vi "SubPanel_PowerConfiguration_Rev11.vi"(8 "error in":errorcluster, 10 "VISAPowerInfoInputArray":T1(array[cluster]), 11 "DCPowerInformationClusterArray_Input":T3(array[cluster])) -> (0 "error out":errorcluster, 2 "VISAPowerInfoOutputArray":T1(array[cluster]), 3 "DCPowerInformationClusterArray_Output":T3(array[cluster]))   [LabVIEW 2019]
panel:
  out "VISAPowerInformationClusterArray":T1(array[cluster])
  out "DCPowerInformationClusterArray":T2(array[cluster])
  out "VISAPowerInformationClusterOutput":T4(array[cluster])
  in  "VISAPowerInformationClusterInput":T4(array[cluster])
  in  "Exit SubVI":bool
  in  "Instrument Cards (Must Reconfigure if you add new cards or change the names in NI Max)":T5(tab)=enum."PXIe-4139"
  in  "VISA resource name":refnum<visa-resource-name>
  in  "Apply Power Settings":bool
  out "POWER STATUS":bool
  in  "POWER ON":bool
  in  "Voltage Channel 1":dbl
  in  "Voltage Channel 2":dbl
  in  "Voltage Channel 3":dbl
  in  "Current Limit Channel 1":dbl
  in  "Current Limit Channel 2":dbl
  in  "Current Limit Channel 3":dbl
  out "Parameter Configuration Echo":string[][](array[string])
  out "Configuration Echo":string
  in  "Which Channels to Parallelize":u16(ring) items=["I1+I2", "ALL", "I2+I3"]
  in  "Combination Scheme":u16(ring) items=["OFF", "SERIES", "PARALLEL"]
  in  "voltage level channel 0":dbl format="%.6p"
  in  "voltage level channel 1":dbl format="%.6p"
  in  "voltage level channel 2":dbl format="%.6p"
  in  "voltage level channel 3":dbl format="%.6p"
  in  "voltage level channel 4":dbl format="%.6p"
  in  "voltage level channel 5":dbl format="%.6p"
  in  "voltage level channel 6":dbl format="%.6p"
  in  "voltage level channel 7":dbl format="%.6p"
  in  "voltage level channel 8":dbl format="%.6p"
  in  "voltage level channel 9":dbl format="%.6p"
  in  "voltage level channel 10":dbl format="%.6p"
  in  "voltage level channel 11":dbl format="%.6p"
  in  "voltage level channel 12":dbl format="%.6p"
  in  "voltage level channel 13":dbl format="%.6p"
  in  "voltage level channel 14":dbl format="%.6p"
  in  "voltage level channel 15":dbl format="%.6p"
  in  "voltage level channel 16":dbl format="%.6p"
  in  "voltage level channel 17":dbl format="%.6p"
  in  "voltage level channel 18":dbl format="%.6p"
  in  "voltage level channel 19":dbl format="%.6p"
  in  "voltage level channel 20":dbl format="%.6p"
  in  "voltage level channel 21":dbl format="%.6p"
  in  "voltage level channel 22":dbl format="%.6p"
  in  "voltage level channel 23":dbl format="%.6p"
  in  "Active Channel 0":bool
  in  "Active Channel 1":bool
  in  "Active Channel 2":bool
  in  "Active Channel 3":bool
  in  "Active Channel 4":bool
  in  "Active Channel 5":bool
  in  "Active Channel 6":bool
  in  "Active Channel 7":bool
  in  "Active Channel 8":bool
  in  "Active Channel 9":bool
  in  "Active Channel 10":bool
  in  "Active Channel 11":bool
  in  "Active Channel 12":bool
  in  "Active Channel 13":bool
  in  "Active Channel 14":bool
  in  "Active Channel 15":bool
  in  "Active Channel 16":bool
  in  "Active Channel 17":bool
  in  "Active Channel 18":bool
  in  "Active Channel 19":bool
  in  "Active Channel 20":bool
  in  "Active Channel 21":bool
  in  "Active Channel 22":bool
  in  "Active Channel 23":bool
  in  "Channel Name 0":string="NULL0"
  in  "Channel Name 1":string="1p8V_supply"
  in  "Channel Name 2":string="NULL2"
  in  "Channel Name 3":string="NULL3"
  in  "Channel Name 4":string="NULL4"
  in  "Channel Name 5":string="NULL5"
  in  "Channel Name 6":string="NULL6"
  in  "Channel Name 7":string="NULL7"
  in  "Channel Name 8":string="NULL8"
  in  "Channel Name 9":string="NULL9"
  in  "Channel Name 10":string="NULL10"
  in  "Channel Name 11":string="NULL11"
  in  "Channel Name 12":string="NULL12"
  in  "Channel Name 13":string="NULL13"
  in  "Channel Name 14":string="NULL14"
  in  "Channel Name 15":string="NULL15"
  in  "Channel Name 16":string="NULL16"
  in  "Channel Name 17":string="NULL17"
  in  "Channel Name 18":string="NULL18"
  in  "Channel Name 19":string="NULL19"
  in  "Channel Name 20":string="NULL20"
  in  "Channel Name 21":string="NULL21"
  in  "Channel Name 22":string="NULL22"
  in  "Channel Name 23":string="NULL23"
  in  "Apply Power Settings":bool
  in  "Aperture Time (s)":dbl=0.0001
  in  "Measure Record Length":i32=1000000
  in  "current limit (A)":dbl=0.05
  out "All Channel Numbers Array":string[](array[string])=["0", "1", "2", "3", "4", "5", "6", "7", "8", "9", "10", "11", "12", "13", "14", "15", "16", "17", "18", "19", "20", "21", "22", "23"]
  out "Active Channels Indicator":bool[](array[boolean])
  out "Voltage Array":dbl[](array[numeric])=[1.0, 1.8, 1.2, 1.3, 1.4, 1.5, 1.6, 1.7, 1.8, 1.9, 2.0, 2.1, 2.2, 2.3, 2.4, 2.5, 2.6, 2.7, 2.8, 2.9, 3.0, 3.1, 3.2, 3.3]
  out "Active Channel Numbers Array":string[](array[string])=["1"]
  out "Active Channel Voltage Array":dbl[](array[numeric])=[1.8]
  out "Active Channel Names Array":string[](array[string])=["1p8V_supply"]
  in  "voltage level channel 0":dbl format="%.6p"
  in  "Active Channel 0":bool
  in  "Apply Power Settings":bool
  in  "Channel Name 0":string="1p6_supply"
  out "Active Channel Voltage Array":dbl[](array[numeric])=[1.68]
  out "Active Channels Indicator":bool[](array[boolean])
  out "Voltage Array":dbl[](array[numeric])=[1.68]
  out "Active Channel Names Array":string[](array[string])=["1p6_supply"]
  out "Active Channel Numbers Array":string[](array[string])=["0"]
  out "All Channel Numbers Array":string[](array[string])=["0"]
  in  "current limit (A)":dbl=0.05
  in  "Measure Record Length":i32=1000000
  in  "Aperture Time (s)":dbl=0.001
  out "DCPowerInformationClusterOutput":T6(array[cluster])
  in  "DCPowerInformationClusterInput":T6(array[cluster])
  # "Background Information (Important)\nThis subvi has tabs that allow you to configure different power instruments. There are two options: VISA instruments or DC Power instruments. DC Power instruments are inside of the tester, visa instruments are external. If DCPower instruments are switched out, they will need to be reconfigured within the backend of this code (instructions pending). You are able to identify which channels you want to active, their individual voltage levels and the desired \"name\" of the channel (i.e. if you want channel 0 to be known at the \"ADMV1013_3p3V\" or \"GoodEnough\", you write it here). For the entire instrument, you can determine its capture rate (aperture time) or the current limit. I advise you do NOT alter the \"Measure Record Length\" as this is only if there are issues with the program. Shouldn't ever exceed this value. You apply the settings and they will be echoed back in each tab along with the array above. Multiple instruments can be configured and will show up as separate array elements\n\n\nInstructions (More Important):\n\nSelect instrument of interest (VISA KEITHLEY 2230G-30-6, PXIe-4163, and PXIe-4139 are the ones currently available). \n\n\nFOR DCPOWER INSTRUMENTS (PXI or PXIe)\n\nPress \"Active Channel #\" to select which channels you want to have power applied \n\nType in voltage level in \"Voltage level channel #\"\n\nType in desired channel name in \"Channel Name #\"\n\nType the measurement speed (suggest .0001) in aperture time\n\nType the current limit in \"current limit\"\n\nPress \"Apply Power Settings\" and review the echoed outputs within the tab and in the instrument array above the tabs.\n\nRepeat this process for other instruments\n\n\n\nFOR VISA INSTRUMENTS (NOT PXI or PXIe), note that it is case by case for instruments\n\nSelect resource name (you must know which one it is)\n\nPower on device if using it\n\nApply voltage settings \n\nApply current limits for each channel\n\nSelect which channels you will parallelize if at all\n\nSelect which combination scheme you will apply: OFF (individual channels), SERIES (Channel 1 and 2 in series), PARALLEL (I1 + I2, ALL, I2 + I3)\n\nFOR COMBINATIONS: for a combination scheme you choose, you only apply changes to the first channel of each. example: if you make the system series configuration, you only type you voltage information (i.e. 60V) into channel 1 and the current limit information into channel 1 but channel 3 is still independent of these\n\n\nPress \"Apply Powe Settings\" when complete\n\nReview the echoed values along with the instrument array above"
  # "All Voltage Level Channels are in Volts"
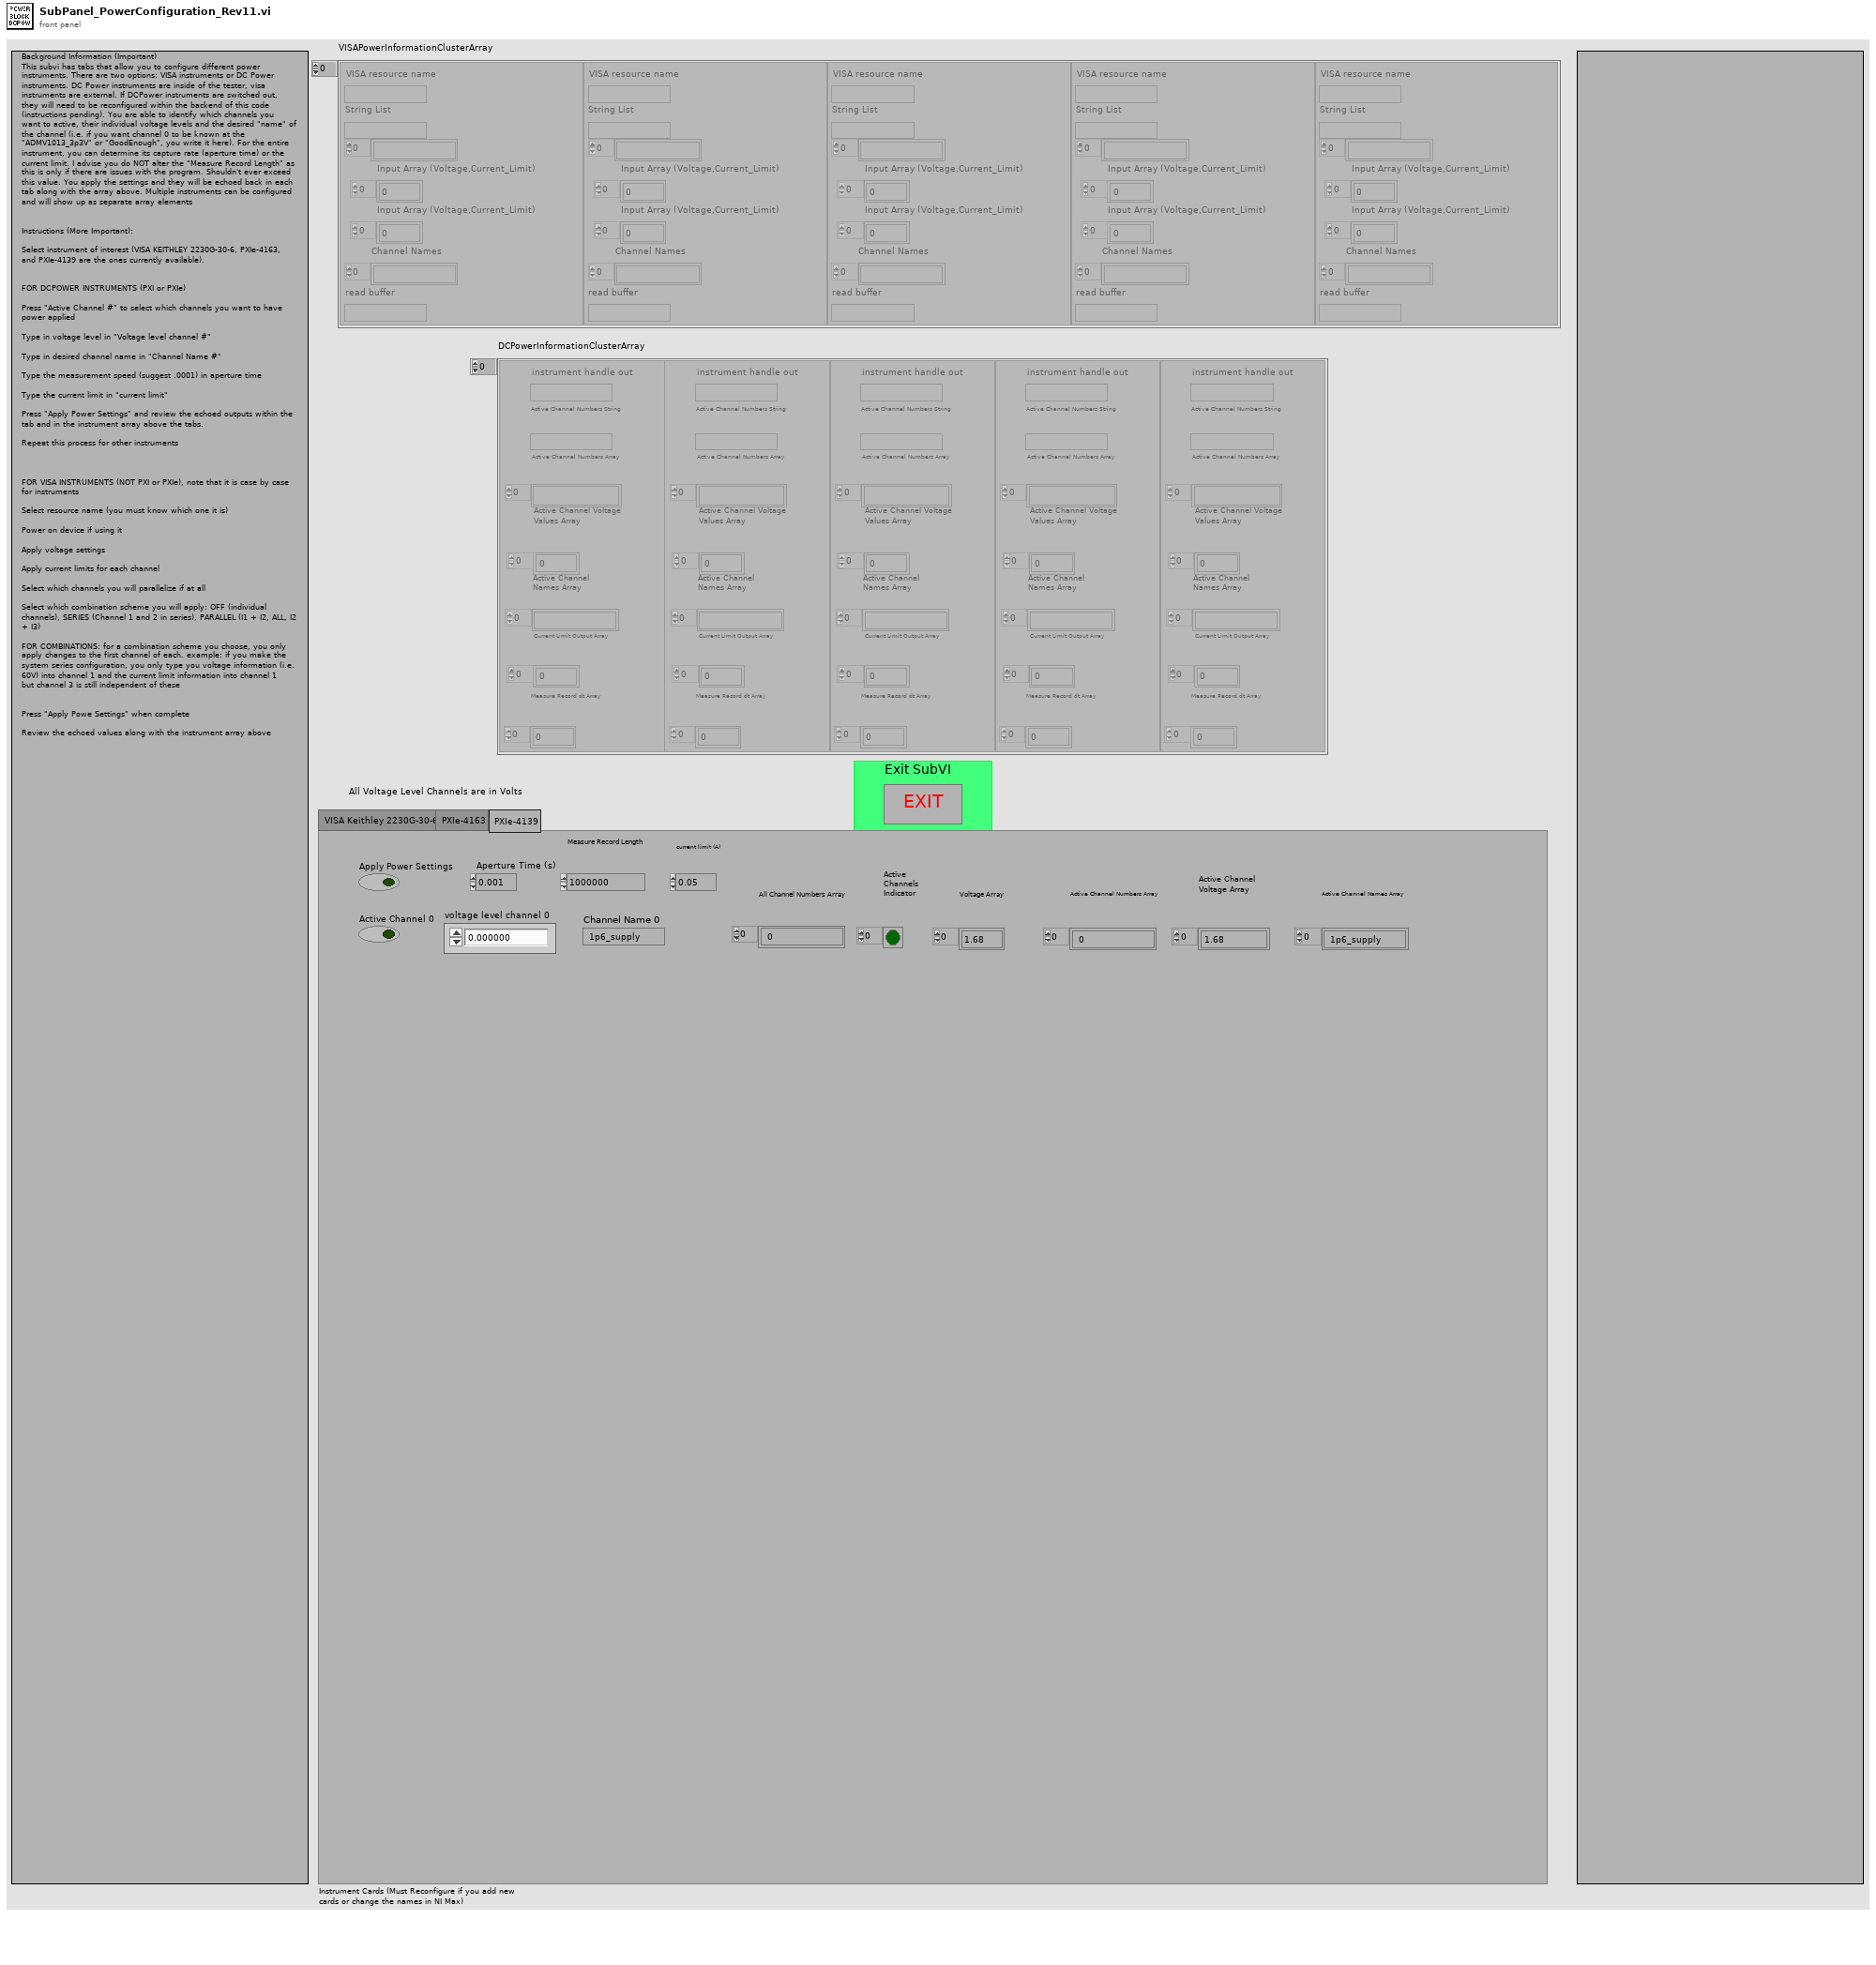
[diagram p1: front panel]
types:
  T1 = cluster{"VISA resource name":refnum<visa-resource-name>, "String List":string, string[], "Input Array (Voltage,Current_Limit)":dbl[], "Input Array (Voltage,Current_Limit)":dbl[], "Channel Names":string[], "read buffer":string}[]
  T2 = cluster{"instrument handle out":refnum<k15>, "Active Channel Numbers String":string, "Active Channel Numbers Array":string[], "Active Channel Voltage Values Array":dbl[], "Active Channel Names Array":string[], "Current Limit Output Array":dbl[], "Measure Record dt Array":dbl[]}[]
  T3 = cluster{"instrument handle out":refnum<k15>, string, string[], dbl[], string[], "Current Limit Output Array":dbl[], dbl[]}[]
  T4 = cluster{"VISA resource name":refnum<visa-resource-name>, "String List":string, string[], "Input Array (Voltage,Current_Limit)":dbl[], "Input Array (Voltage,Current_Limit)":dbl[], "Channel Names":string[]}[]
  T5 = enum32{"VISA Keithley 2230G-30-6", "PXIe-4163", "PXIe-4139"}
  T6 = cluster{"instrument handle out":refnum<k15>, string, string[], dbl[], string[]}[]
  T7 = cluster{"IVI Refnum out":refnum<k15>, "Active Channel Numbers String List":string, "Active Channel Numbers Array":string[], "Active Channel Voltage Array":dbl[], "Active Channel Names Array":string[], "Active Channel Current Limit Array":dbl[], "Active Channel Measure Record Delta Time Array":dbl[]}
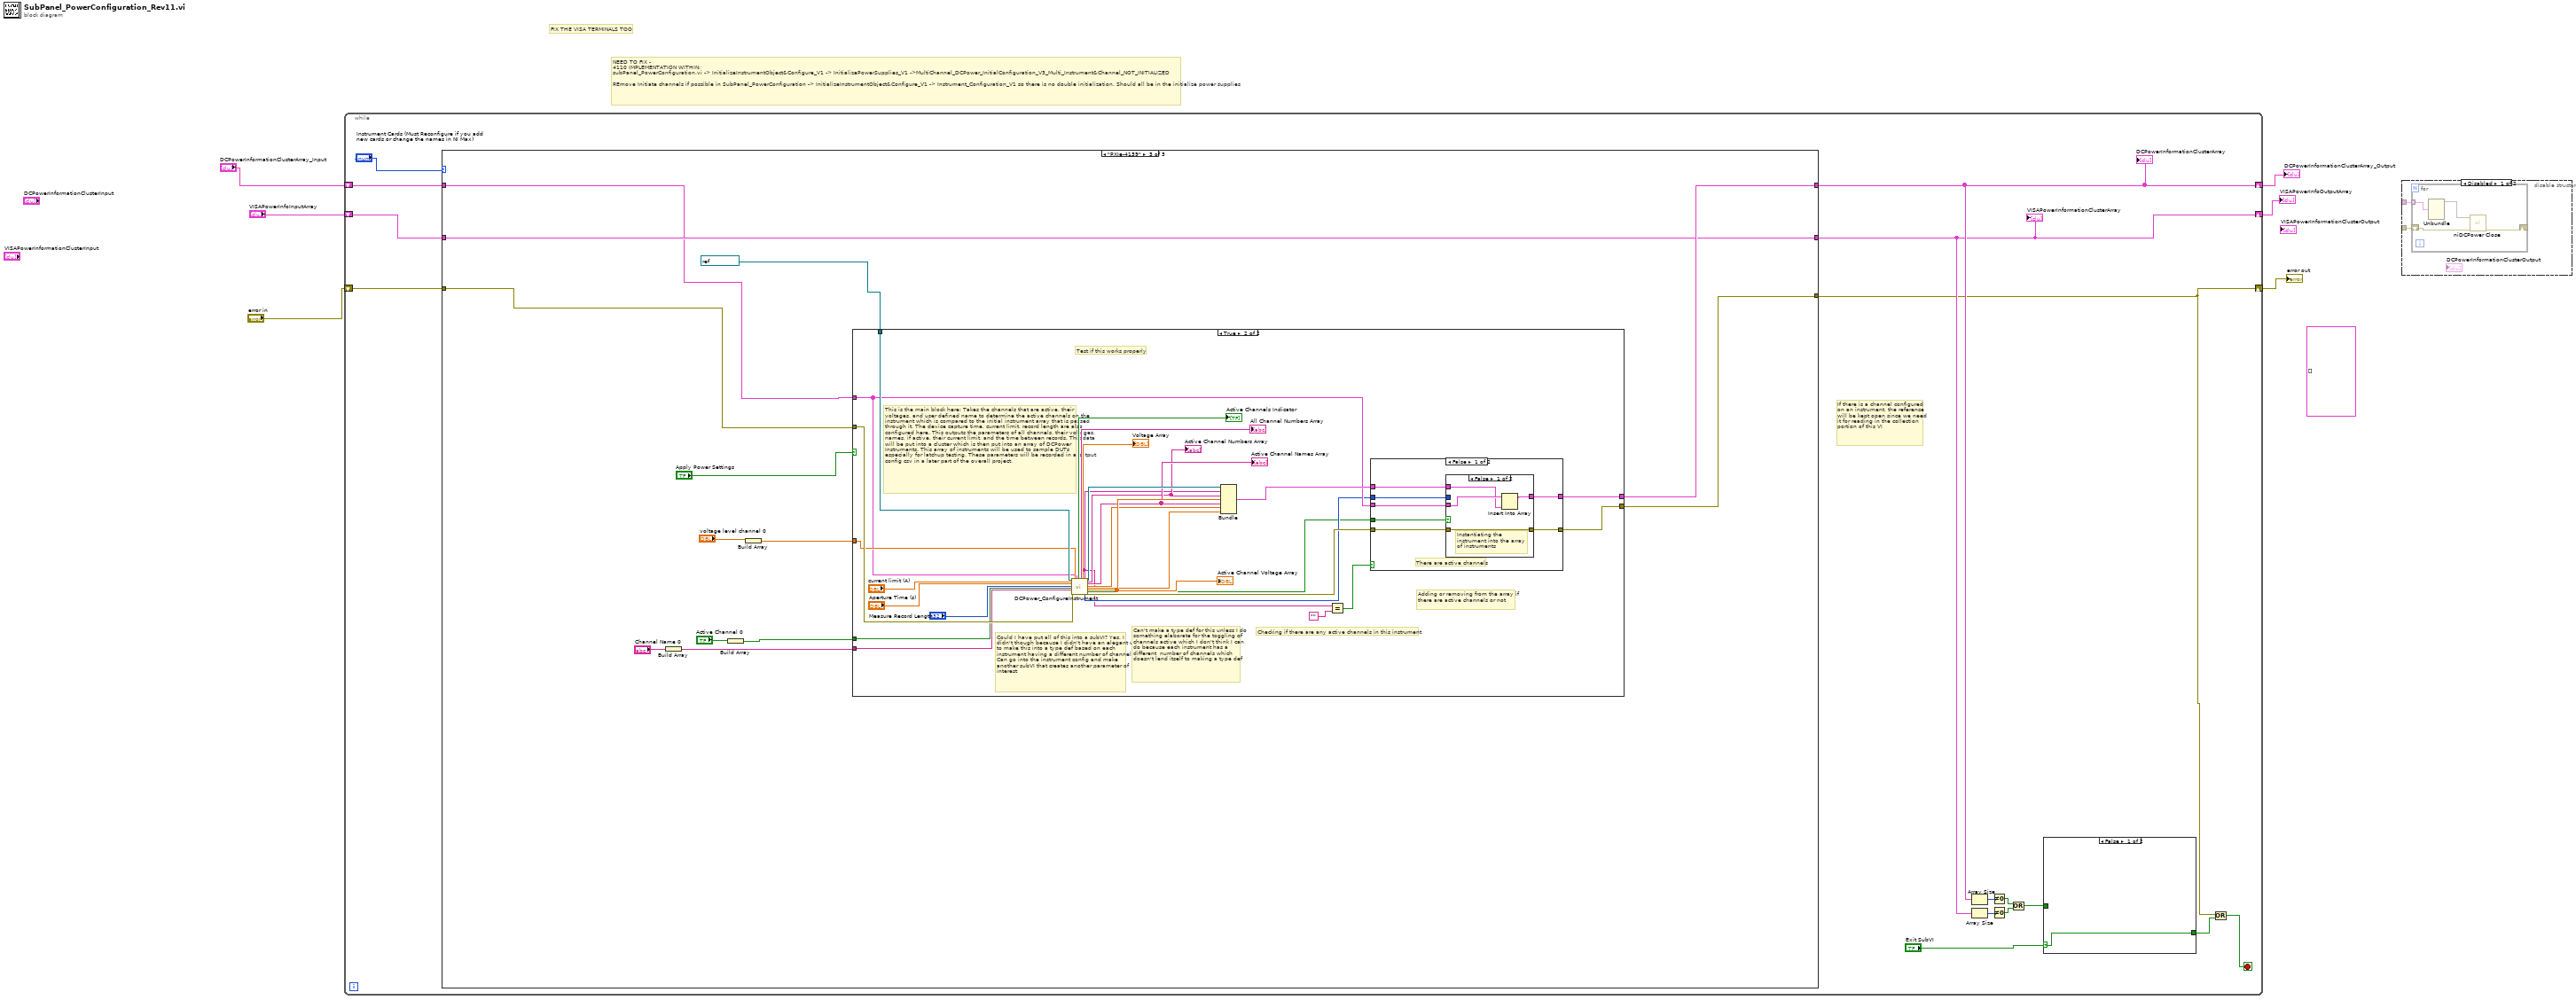
[diagram p0: block diagram]
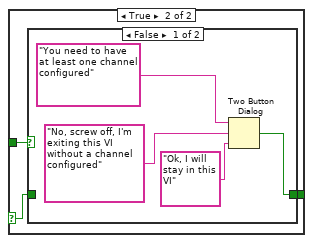
[diagram p3: hidden frame]
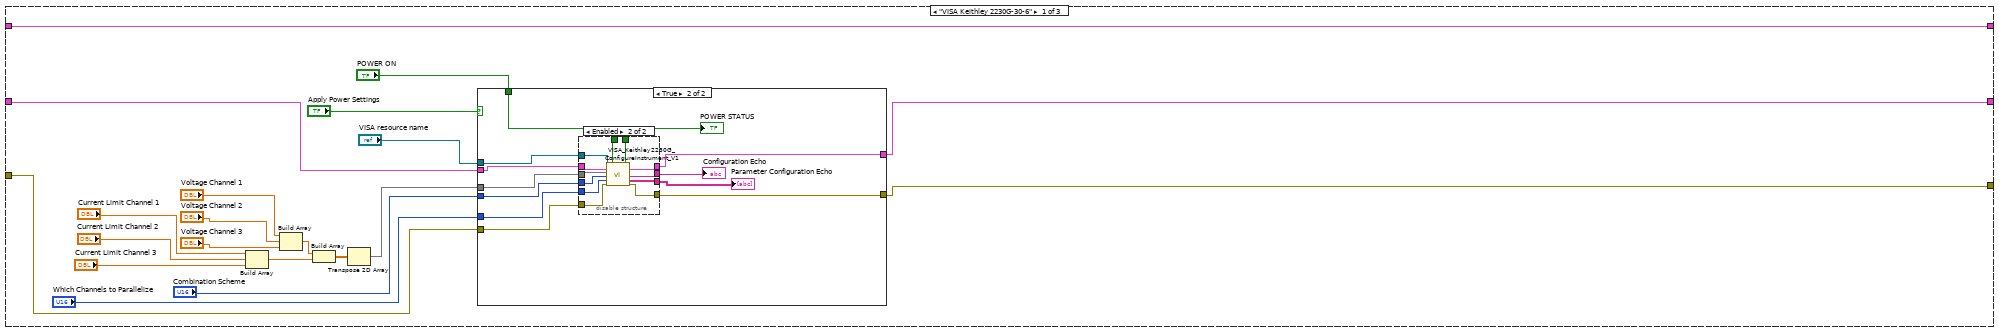
[diagram p5: hidden frame]
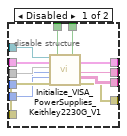
[diagram p7: hidden frame]
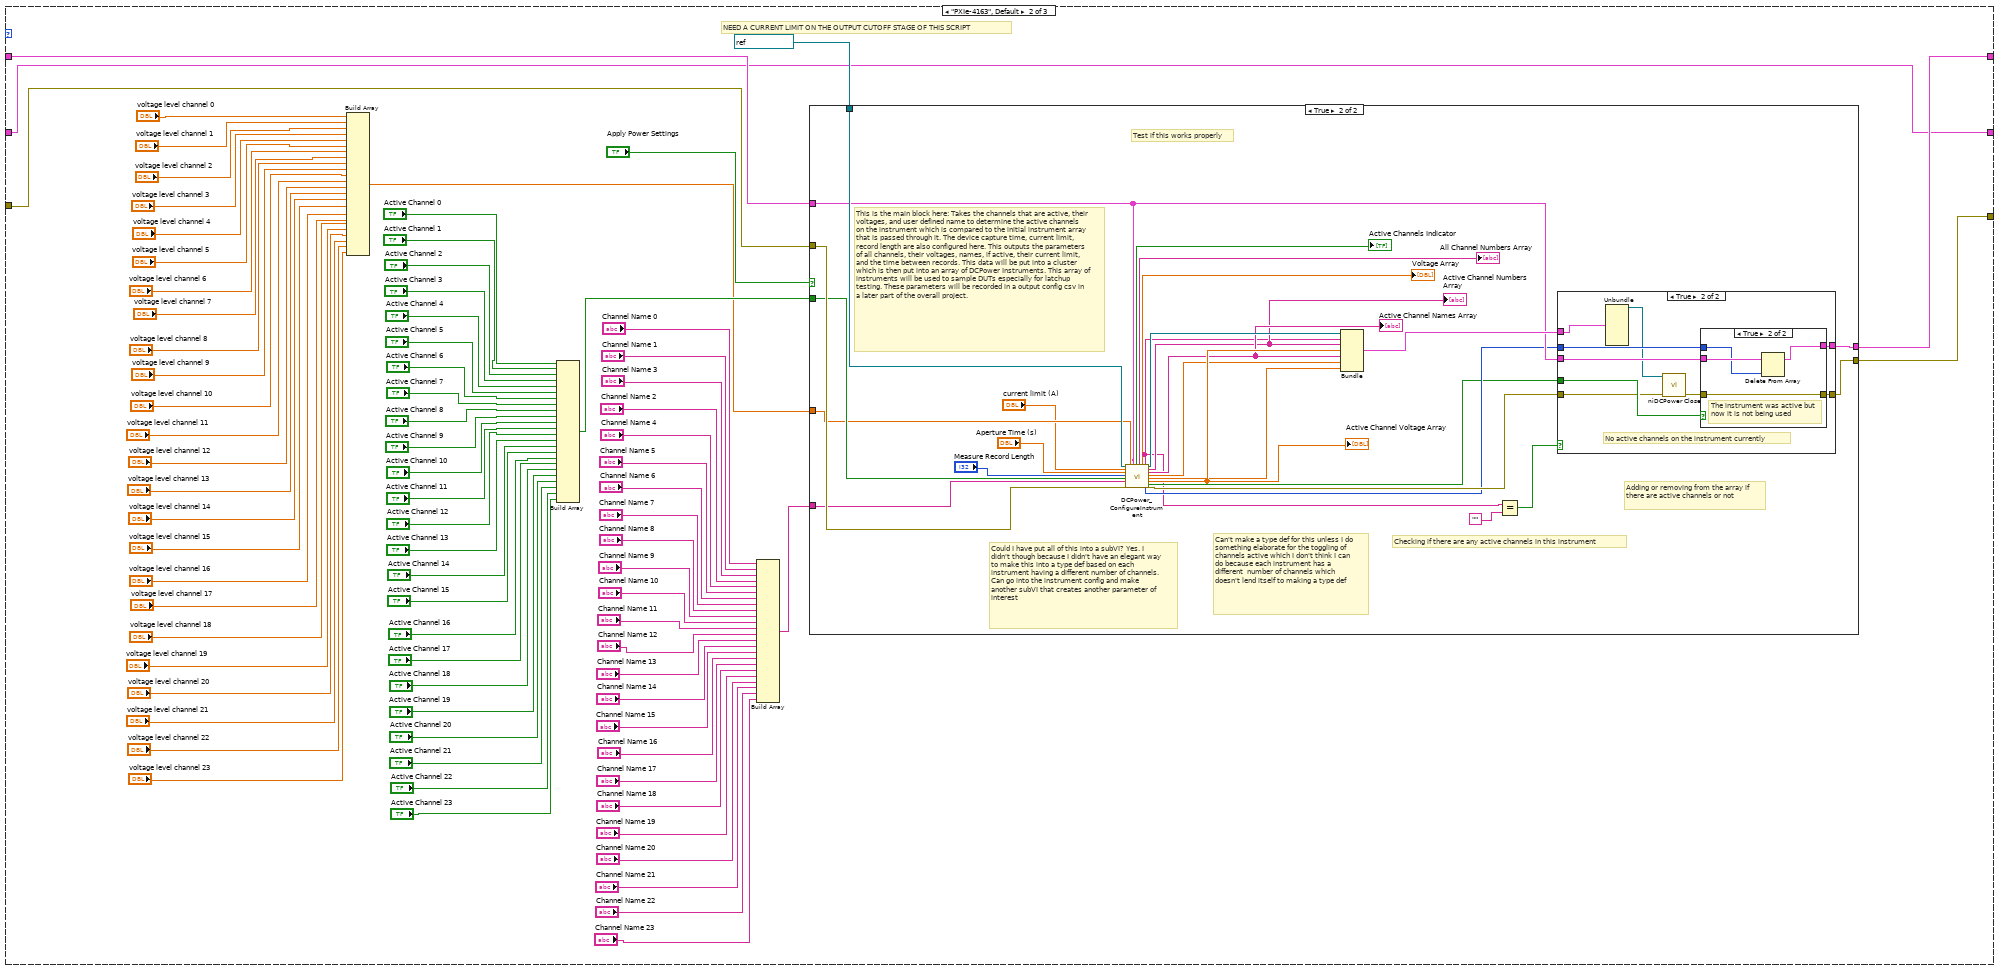
[diagram p8: hidden frame]
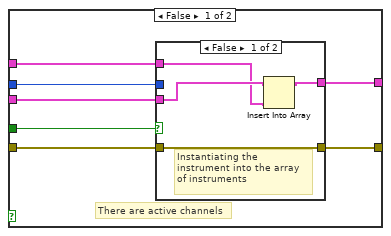
[diagram p10: hidden frame]
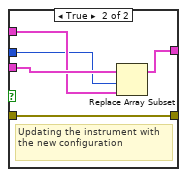
[diagram p11: hidden frame]
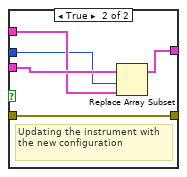
[diagram p14: hidden frame]
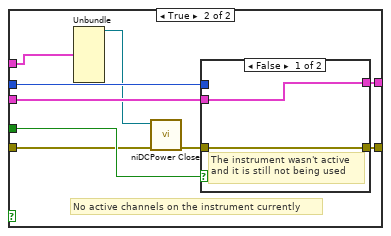
[diagram p15: hidden frame]
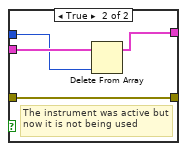
[diagram p16: hidden frame]
diagram:
  (unwired) T3 [] ("DCPowerInformationClusterArray_Input")
  # "FIX THE VISA TERMINALS TOO"
  # "NEED TO FIX - \n4110 IMPLEMENTATION WITHIN:\nsubPanel_PowerConfiguration.vi -> InitializeInstrumentObject&Configure_V1 -> InitializePowerSupplies_V1 ->MultiChannel_DCPower_InitialConfiguration_V3_Multi_Instrument&Channel_NOT_INITIALIZED\n\nREmove Initiate channels if possible in SubPanel_PowerConfiguration -> InitializeInstrumentObject&Configure_V1 -> Instrument_Configuration_V1 so there is no double initialization. Should all be in the initialize power supplies"
  n1 = while {
    shift-right: [w17] -> w1
    shift-left: "DCPowerInformationClusterArray_Input" -> [w21]
    shift-right: [w9] -> w5
    shift-left: "error in" -> [w20]
    shift-right: [w16] -> w3
    shift-left: "VISAPowerInfoInputArray" -> [w18]
    stop <- w7 stop-if-true
    # "If there is a channel configured on an instrument, the reference will be kept open since we need it for reading in the collection portion of this VI"
    n2 = case shown="\"PXIe-4139\"" "Instrument Cards (Must Reconfigure if you add new cards or change the names in NI Max)" {
      tunnel: w21 -> [w47 w97 w231]
      tunnel: w20 -> [w35 w93 w239]
      tunnel: [w32 w92 w233] -> w9
      tunnel: [w47 w91 w234] -> w17
      tunnel: w18 -> [w48 w90 w232]
      tunnel: [w31 w90 w232] -> w16
      frame "VISA Keithley 2230G-30-6" {
        n3 = Build Array("Current Limit Channel 1", "Current Limit Channel 2", "Current Limit Channel 3") -> (w45:dbl[])
        n4 = Build Array("Voltage Channel 1", "Voltage Channel 2", "Voltage Channel 3") -> (w44:dbl[])
        n5 = Build Array(w44, w45) -> (w46:dbl[][])
        n6 = Transpose 2D Array(2D array=w46) -> (transposed array=w36:dbl[][])
        n7 = case shown="True" "Apply Power Settings" {
          tunnel: "VISA resource name" -> [_ w64]
          tunnel: w48 -> [w51 w63]
          tunnel: "POWER ON" -> [_ w62]
          tunnel: w36 -> [_ w61]
          tunnel: w35 -> [w52 w60]
          tunnel: "Which Channels to Parallelize" -> [_ w59]
          tunnel: "Combination Scheme" -> [_ w58]
          tunnel: [w51 w54] -> w31
          tunnel: [w52 w53] -> w32
          frame False {
          }
          frame True {
            n8 = disable-structure shown="Enabled" {
              disable-tunnel: w64 -> [w76 w86]
              disable-tunnel: w63 -> [w75 w85]
              disable-tunnel: w62 -> [w74 w87]
              disable-tunnel: w61 -> [w73 w84]
              disable-tunnel: w60 -> [w72 w81]
              disable-tunnel: w59 -> [w71 w82]
              disable-tunnel: w58 -> [w70 w83]
              disable-tunnel: [w69 w88] -> w57
              disable-tunnel: [w68 w79] -> w56
              disable-tunnel: [w67 w78] -> w55
              disable-tunnel: [w66 w80] -> w54
              disable-tunnel: [w65 w77] -> w53
              frame Disabled {
                n9 = call "Initialize_VISA_PowerSupplies_Keithley2230G_V1.vi"("VISA resource name"=w76, "VISAPowerInfoInputArray"=w75, "Input Array (Voltage,Current_Limit)"=w73, "Combination Scheme"=w70, "Which Channels to Parallelize"=w71, "error in"=w72, "POWER STATUS IN"=w74) -> ("POWER STATUS OUT"=w69:bool, "VISAPowerInfoOutputArray"=w66:T1, "Configuration Echo"=w68:string, "Parameter Configuration Echo"=w67:string[][], "error out"=w65:errorcluster)  [unwired: 8 in]
              }
              frame Enabled {
                n10 = call "VISA_Keithley2230G_ConfigureInstrument_V1.vi"("VISA resource name"=w86, "VISAPowerInfoInputArray"=w85, "Input Array (Voltage,Current_Limit)"=w84, "Combination Scheme"=w83, "Which Channels to Parallelize"=w82, "error in"=w81, "POWER STATUS IN"=w87) -> ("POWER STATUS OUT"=w88:bool, "VISAPowerInfoOutputArray"=w80:T1, "Configuration Echo"=w79:string, "Parameter Configuration Echo"=w78:string[][], "error out"=w77:errorcluster)  [unwired: 8 in]
              }
            }
            "POWER STATUS" <- w57
            "Configuration Echo" <- w56
            "Parameter Configuration Echo" <- w55
          }
        }
      }
      frame "PXIe-4163", Default {
        # "NEED A CURRENT LIMIT ON THE OUTPUT CUTOFF STAGE OF THIS SCRIPT"
        n11 = Build Array("voltage level channel 0", "voltage level channel 1", "voltage level channel 2", "voltage level channel 3", "voltage level channel 4", "voltage level channel 5", "voltage level channel 6", "voltage level channel 7", "voltage level channel 8", "voltage level channel 9", "voltage level channel 10", "voltage level channel 11", "voltage level channel 12", "voltage level channel 13", "voltage level channel 14", "voltage level channel 15", "voltage level channel 16", "voltage level channel 17", "voltage level channel 18", "voltage level channel 19", "voltage level channel 20", "voltage level channel 21", "voltage level channel 22", "voltage level channel 23") -> (w89:dbl[])
        n12 = Build Array("Active Channel 0", "Active Channel 1", "Active Channel 2", "Active Channel 3", "Active Channel 4", "Active Channel 5", "Active Channel 6", "Active Channel 7", "Active Channel 8", "Active Channel 9", "Active Channel 10", "Active Channel 11", "Active Channel 12", "Active Channel 13", "Active Channel 14", "Active Channel 15", "Active Channel 16", "Active Channel 17", "Active Channel 18", "Active Channel 19", "Active Channel 20", "Active Channel 21", "Active Channel 22", "Active Channel 23") -> (w95:bool[])
        n13 = Build Array("Channel Name 0", "Channel Name 1", "Channel Name 3", "Channel Name 2", "Channel Name 4", "Channel Name 5", "Channel Name 6", "Channel Name 7", "Channel Name 8", "Channel Name 9", "Channel Name 10", "Channel Name 11", "Channel Name 12", "Channel Name 13", "Channel Name 14", "Channel Name 15", "Channel Name 16", "Channel Name 17", "Channel Name 18", "Channel Name 19", "Channel Name 20", "Channel Name 21", "Channel Name 22", "Channel Name 23") -> (w94:string[])
        n14 = case shown="True" "Apply Power Settings" {
          tunnel: w97 -> [w172 w181]
          tunnel: refnum<k15> "PXIe-4163" ("resource name") -> [_ w199]
          tunnel: w95 -> [_ w197]
          tunnel: w94 -> [_ w195]
          tunnel: w93 -> [w171 w198]
          tunnel: [w171 w179] -> w92
          tunnel: [w172 w178] -> w91
          tunnel: w89 -> [_ w196]
          frame False {
          }
          frame True {
            # "This is the main block here: Takes the channels that are active, their voltages, and user defined name to determine the active channels on the instrument which is compared to the initial instrument array that is passed through it. The device capture time, current limit, record length are also configured here. This outputs the parameters of all channels, their voltages, names, if active, their current limit, and the time between records. This data will be put into a cluster which is then put into an array of DCPower Instruments. This array of instruments will be used to sample DUTs especially for latchup testing. These parameters will be recorded in a output config csv in a later part of the overall project."
            # "Checking if there are any active channels in this instrument"
            # "Adding or removing from the array if there are active channels or not"
            # "Could I have put all of this into a subVI? Yes. I didn't though because I didn't have an elegant way to make this into a type def based on each instrument having a different number of channels. Can go into the instrument config and make another subVI that creates another parameter of interest"
            # "Can't make a type def for this unless I do something elaborate for the toggling of channels active which I don't think I can do because each instrument has a different  number of channels which doesn't lend itself to making a type def"
            # "Test if this works properly"
            n15 = call "DCPower_ConfigureInstrument.vi"("IVI Refnum in"=w199, "current limit"="current limit (A)", "Aperture Time"="Aperture Time (s)", "Measure Record Length"="Measure Record Length", "Active Channels Input"=w197, "Channel Name Array"=w195, "error in (no error)"=w198, "Voltage Array Input"=w196, "DCPowerInformationClusterArray_Input"=w181) -> ("Active Channels Indicator"=→"Active Channels Indicator":bool[], "All Channel Numbers Array"=→"All Channel Numbers Array":string[], "Total Voltage Indicator Array"=→"Voltage Array":dbl[], "Active Channel Numbers String List"=w173:string, "IVI Ref index"=w177:i32, "IVI Refnum out"=w190:refnum<k15>, "Active Channel Numbers Array"=w175:string[], "Active Channel Names Array"=w187:string[], "Active Channel Current Limit Array"=w186:dbl[], "Active Channel Measure Record Delta Time Array"=w185:dbl[], "Active Channel Voltage Array"=w188:dbl[], "IVI Ref Present?"=w176:bool, "error out"=w180:errorcluster)  [unwired: 5 in, 1 out]
            "Active Channel Numbers Array" <- w175
            "Active Channel Names Array" <- w187
            "Active Channel Voltage Array" <- w188
            n16 = Bundle("IVI Refnum out"=w190, "Active Channel Numbers String List"=w173, "Active Channel Numbers Array"=w175, "Active Channel Voltage Array"=w188, "Active Channel Names Array"=w187, "Active Channel Current Limit Array"=w186, "Active Channel Measure Record Delta Time Array"=w185) -> (w182:T7)  [unwired: 1 in]
            n17 = Equal?(x=w173, y="") -> (x = y?=w183:bool)
            n18 = case shown="True" w183 {
              tunnel: w176 -> [w206 w223]
              tunnel: [w205 w220] -> w178
              tunnel: [w204 w221] -> w179
              tunnel: w180 -> [w203 w218]
              tunnel: w177 -> [w202 w222]
              tunnel: w182 -> [w201 w216]
              tunnel: w181 -> [w200 w224]
              frame False {
                # "There are active channels"
                n19 = case shown="False" w206 {
                  tunnel: w200 -> [w209 w215]
                  tunnel: w201 -> [w208 w214]
                  tunnel: w202 -> [_ w213]
                  tunnel: w203 -> [w210 w212]
                  tunnel: [w210 w212] -> w204
                  tunnel: [w207 w211] -> w205
                  frame False {
                    # "Instantiating the instrument into the array of instruments"
                    n20 = Insert Into Array(array=w209, new element=w208) -> (w207:T3)  [unwired: 1 in]
                  }
                  frame True {
                    # "Updating the instrument with the new configuration"
                    n21 = Replace Array Subset(array=w215, new element=w214, index=w213) -> (w211:T3)
                  }
                }
              }
              frame True {
                # "No active channels on the instrument currently"
                n22 = Unbundle(w216) -> ("IVI Refnum out"=w219:refnum<k15>)  [unwired: 6 out]
                n23 = call <instrlib>:"niDCPower Close.vi"("error in (no error)"=w218, "instrument handle"=w219) -> ("error out"=w217:errorcluster)  [unwired: 9 in]
                n24 = case shown="True" w223 {
                  tunnel: w224 -> [w226 w230]
                  tunnel: w222 -> [_ w229]
                  tunnel: [w225 w228] -> w221
                  tunnel: w217 -> [w225 w228]
                  tunnel: [w226 w227] -> w220
                  frame False {
                    # "The instrument wasn't active and it is still not being used"
                  }
                  frame True {
                    # "The instrument was active but now it is not being used"
                    n25 = Delete From Array(array=w230, index=w229) -> (array with subset deleted=w227:T3)  [unwired: 1 in, 1 out]
                  }
                }
              }
            }
          }
        }
      }
      frame "PXIe-4139" {
        n26 = Build Array("Channel Name 0") -> (w236:string[])
        n27 = Build Array("Active Channel 0") -> (w237:bool[])
        n28 = Build Array("voltage level channel 0") -> (w238:dbl[])
        n29 = case shown="True" "Apply Power Settings" {
          tunnel: w231 -> [w245 w254]
          tunnel: refnum<k15> "PXI-4139" ("resource name") -> [_ w272]
          tunnel: w237 -> [_ w270]
          tunnel: w236 -> [_ w268]
          tunnel: w239 -> [w244 w271]
          tunnel: [w244 w252] -> w233
          tunnel: [w245 w251] -> w234
          tunnel: w238 -> [_ w269]
          frame False {
          }
          frame True {
            # "This is the main block here: Takes the channels that are active, their voltages, and user defined name to determine the active channels on the instrument which is compared to the initial instrument array that is passed through it. The device capture time, current limit, record length are also configured here. This outputs the parameters of all channels, their voltages, names, if active, their current limit, and the time between records. This data will be put into a cluster which is then put into an array of DCPower Instruments. This array of instruments will be used to sample DUTs especially for latchup testing. These parameters will be recorded in a output config csv in a later part of the overall project."
            # "Checking if there are any active channels in this instrument"
            # "Adding or removing from the array if there are active channels or not"
            # "Could I have put all of this into a subVI? Yes. I didn't though because I didn't have an elegant way to make this into a type def based on each instrument having a different number of channels. Can go into the instrument config and make another subVI that creates another parameter of interest"
            # "Can't make a type def for this unless I do something elaborate for the toggling of channels active which I don't think I can do because each instrument has a different  number of channels which doesn't lend itself to making a type def"
            # "Test if this works properly"
            n30 = call "DCPower_ConfigureInstrument.vi"("IVI Refnum in"=w272, "current limit"="current limit (A)", "Aperture Time"="Aperture Time (s)", "Measure Record Length"="Measure Record Length", "Active Channels Input"=w270, "Channel Name Array"=w268, "error in (no error)"=w271, "Voltage Array Input"=w269, "DCPowerInformationClusterArray_Input"=w254) -> ("Active Channels Indicator"=→"Active Channels Indicator":bool[], "All Channel Numbers Array"=→"All Channel Numbers Array":string[], "Total Voltage Indicator Array"=→"Voltage Array":dbl[], "Active Channel Numbers String List"=w246:string, "IVI Ref index"=w250:i32, "IVI Refnum out"=w263:refnum<k15>, "Active Channel Numbers Array"=w248:string[], "Active Channel Names Array"=w260:string[], "Active Channel Current Limit Array"=w259:dbl[], "Active Channel Measure Record Delta Time Array"=w258:dbl[], "Active Channel Voltage Array"=w261:dbl[], "IVI Ref Present?"=w249:bool, "error out"=w253:errorcluster)  [unwired: 5 in, 1 out]
            "Active Channel Numbers Array" <- w248
            "Active Channel Names Array" <- w260
            "Active Channel Voltage Array" <- w261
            n31 = Bundle("IVI Refnum out"=w263, "Active Channel Numbers String List"=w246, "Active Channel Numbers Array"=w248, "Active Channel Voltage Array"=w261, "Active Channel Names Array"=w260, "Active Channel Current Limit Array"=w259, "Active Channel Measure Record Delta Time Array"=w258) -> (w255:T7)  [unwired: 1 in]
            n32 = Equal?(x=w246, y="") -> (x = y?=w256:bool)
            n33 = case shown="False" w256 {
              tunnel: w249 -> [w279 w296]
              tunnel: [w278 w293] -> w251
              tunnel: [w277 w294] -> w252
              tunnel: w253 -> [w276 w291]
              tunnel: w250 -> [w275 w295]
              tunnel: w255 -> [w274 w289]
              tunnel: w254 -> [w273 w297]
              frame False {
                # "There are active channels"
                n34 = case shown="False" w279 {
                  tunnel: w273 -> [w282 w288]
                  tunnel: w274 -> [w281 w287]
                  tunnel: w275 -> [_ w286]
                  tunnel: w276 -> [w283 w285]
                  tunnel: [w283 w285] -> w277
                  tunnel: [w280 w284] -> w278
                  frame False {
                    # "Instantiating the instrument into the array of instruments"
                    n35 = Insert Into Array(array=w282, new element=w281) -> (w280:T3)  [unwired: 1 in]
                  }
                  frame True {
                    # "Updating the instrument with the new configuration"
                    n36 = Replace Array Subset(array=w288, new element=w287, index=w286) -> (w284:T3)
                  }
                }
              }
              frame True {
                # "No active channels on the instrument currently"
                n37 = Unbundle(w289) -> ("IVI Refnum out"=w292:refnum<k15>)  [unwired: 6 out]
                n38 = call <instrlib>:"niDCPower Close.vi"("error in (no error)"=w291, "instrument handle"=w292) -> ("error out"=w290:errorcluster)  [unwired: 9 in]
                n39 = case shown="False" w296 {
                  tunnel: w297 -> [w299 w303]
                  tunnel: w295 -> [_ w302]
                  tunnel: [w298 w301] -> w294
                  tunnel: w290 -> [w298 w301]
                  tunnel: [w299 w300] -> w293
                  frame False {
                    # "The instrument wasn't active and it is still not being used"
                  }
                  frame True {
                    # "The instrument was active but now it is not being used"
                    n40 = Delete From Array(array=w303, index=w302) -> (array with subset deleted=w300:T3)  [unwired: 1 in, 1 out]
                  }
                }
              }
            }
          }
        }
      }
    }
    "DCPowerInformationClusterArray" <- w17
    "VISAPowerInformationClusterArray" <- w16
    n41 = Array Size(array=w17) -> (size(s)=w15:i32)
    n42 = Array Size(array=w16) -> (size(s)=w14:i32)
    n43 = Not Equal To 0?(x=w15) -> (x != 0?=w12:bool)
    n44 = Not Equal To 0?(x=w14) -> (x != 0?=w13:bool)
    n45 = Or(x=w12, y=w13) -> (x .or. y?=w10:bool)
    n46 = case shown="False" "Exit SubVI" {
      selector: "Exit SubVI" -> [w22 w23]
      tunnel: w10 -> [_ w25]
      tunnel: [w22 w24] -> w8
      frame False {
      }
      frame True {
        n47 = case shown="False" w25 {
          tunnel: [w27 w30] -> w24
          tunnel: w23 -> [_ w30]
          frame False {
            n48 = Two Button Dialog(message="You need to have at least one channel configured", 1:"Ok, I will stay in this VI" ("F button name (\"Cancel\")"), 2:"No, screw off, I'm exiting this VI without a channel configured" ("T button name (\"OK\")")) -> (T button?=w27:bool)
          }
          frame True {
          }
        }
      }
    }
    n49 = Or(x=w9, y=w8) -> (x .or. y?=w7:bool)
  }
  "error out" <- w5
  "VISAPowerInfoOutputArray" <- w3
  "DCPowerInformationClusterArray_Output" <- w1
  n50 = disable-structure shown="Disabled" {
    disable-tunnel: _ -> [w305 _]
    disable-tunnel: _ -> [w304 _]
    frame Disabled {
      n51 = for {
        shift-right: [w306] -> _
        shift-left: w305 -> [w309]
        tunnel: w304 -> [w308] mode=indexing
        n52 = Unbundle(w308) -> ("instrument handle out"=w307)  [unwired: 4 out]
        n53 = call <instrlib>:"niDCPower Close.vi"("error in (no error)"=w309, "instrument handle"=w307) -> ("error out"=w306:errorcluster)  [unwired: 9 in]
      }
    }
    frame Enabled {
    }
  }
